vi "Main.vi"() -> ()   [LabVIEW 2013]
uses:
  <vilib>/Utility/sysdir.llb/System Directory Type.ctl
panel:
  out "Application:Kind":T1(ring)
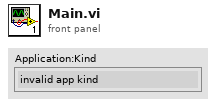
[diagram p1: front panel]
types:
  T1 = enum32{"invalid app kind", "Development System", "Run Time System", "Student Edition", "Embedded LabVIEW", "Evaluation", "Custom"}
  T2 = typedef "System Directory Type.ctl" = i32
  T3 = enum16{"open", "replace", "create", "open or create", "replace or create", "replace or create with confirmation"}
  T4 = cluster{"Missed Shots":dbl, "Over Truss With Catch":dbl, "Over the Truss Pass":dbl, "Defense?":string, "Can they pick up the ball?":string, "Can they catch?":string}
  T5 = cluster{"Autonomous?":string, "Did they start in \nthe goalie zone?":string, "Did they move?":string, "Was the goal lit?":string}
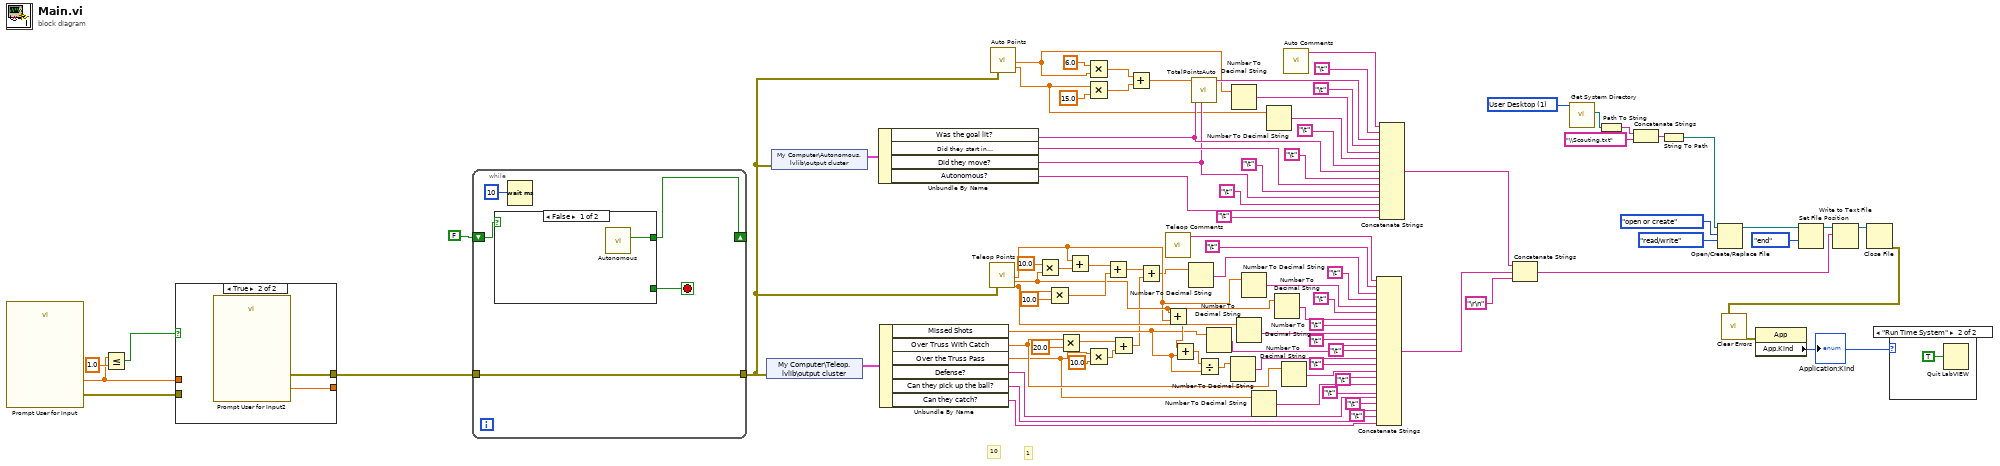
[diagram p0: block diagram]
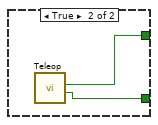
[diagram p4: hidden frame]
diagram:
  w80 = T2 1 items=["User Home"=0, "User Desktop"=1, "User Documents"=2, "User Application Data"=3, "User Preferences"=4, "User Temporary"=5, "Public Documents"=6, "Public Application Data"=7, "Public Preferences"=8, "Public Cache"=13, "System Core Libraries"=9, "System Installed Libraries"=10, "Application Files"=11, "Boot Volume Root"=12] ("system directory type")
  # "1"
  # "10"
  n1 = call "Prompt User for Input"() -> ("Team"=w76:dbl, "error out"=w75:errorcluster)  [unwired: 17 in, 1 out]
  n2 = Less Or Equal?(x=w76, y=1.0 ("x")) -> (x <= y?=w77:bool)
  n3 = case shown="True" w77 {
    tunnel: [w96 w98] -> _
    tunnel: w76 -> [w96 _]
    tunnel: w75 -> [w95 _]
    tunnel: [w95 w97] -> w74
    frame False {
    }
    frame True {
      n4 = call "Prompt User for Input2"() -> ("Team"=w98:dbl, "error out"=w97:errorcluster)  [unwired: 17 in, 1 out]
    }
  }
  n5 = while {
    shift-right: [w101] -> _
    shift-left: FALSE ("Boolean") -> [w102]
    tunnel: w74 -> [w99]
    tunnel: [w99] -> w71
    stop <- w100 stop-if-true
    n6 = case shown="False" w102 {
      tunnel: [w104 w105] -> w101
      tunnel: [_ w106] -> w100
      frame False {
        n7 = call "Autonomous.vi"() -> ("Switch To Teleop"=w104:bool)  [unwired: 10 in, 1 out]
      }
      frame True {
        n8 = call "Teleop.vi"() -> ("Stop program and write to file"=w106:bool, "SWITCH TO AUTONOMOUS 2"=w105:bool)  [unwired: 9 in, 1 out]
      }
    }
    n9 = Wait (ms)(milliseconds to wait=u32 10) -> ()  [unwired: 1 out]
  }
  n10 = shared-variable "My Computer\\Teleop.lvlib\\output cluster"(error in=w71) -> (w73:T4)  [unwired: 1 out]
  n11 = shared-variable "My Computer\\Autonomous.lvlib\\output cluster"(error in=w71) -> (w72:T5)  [unwired: 1 out]
  n12 = Unbundle By Name(w72) -> ("Was the goal lit?"=w58:string, "Did they start in \nthe goalie zone?"=w56:string, "Did they move?"=w54:string, "Autonomous?"=w52:string)
  n13 = Unbundle By Name(w73) -> ("Missed Shots"=w27:dbl, "Over Truss With Catch"=w16:dbl, "Over the Truss Pass"=w13:dbl, "Defense?"=w9:string, "Can they pick up the ball?"=w8:string, "Can they catch?"=w7:string)
  n14 = call "Teleop Points.vi"("Error In"=w71) -> ("Bottom Goal"=w30:dbl, "Top Goal"=w31:dbl, "Assists"=w38:dbl)  [unwired: 15 in, 1 out]
  n15 = call "Auto Points.vi"("Error In"=w71) -> ("Bottom Goal"=w50:dbl, "Top Goal"=w49:dbl)  [unwired: 16 in, 1 out]
  n16 = Multiply(x=10.0, y=w31) -> (x*y=w39:dbl)
  n17 = Multiply(x=w38, y=10.0) -> (x*y=w45:dbl)
  n18 = Multiply(x=w16, y=20.0) -> (x*y=w20:dbl)
  n19 = Add(x=w30, y=w39) -> (x+y=w44:dbl)
  n20 = Multiply(x=6.0, y=w50) -> (x*y=w63:dbl)
  n21 = Multiply(x=w49, y=15.0) -> (x*y=w61:dbl)
  n22 = Multiply(x=w13, y=10.0) -> (x*y=w21:dbl)
  n23 = Add(x=w44, y=w45) -> (x+y=w22:dbl)
  n24 = Add(x=w20, y=w21) -> (x+y=w18:dbl)
  n25 = Add(x=w63, y=w61) -> (x+y=w68:dbl)
  n26 = Add(x=w22, y=w18) -> (x+y=w17:dbl)
  n27 = call "Teleop Comments.vi"() -> ("Teleop Comments"=w48:string)  [unwired: 11 in]
  n28 = Add(x=w31, y=w30) -> (x+y=w29:dbl)
  n29 = Add(x=w29, y=w27) -> (x+y=w28:dbl)
  n30 = Number To Decimal String(number=w17) -> (decimal integer string=w42:string)  [unwired: 1 in]
  n31 = call "TotalPointsAuto.vi"("Did they move?"=w54, "Was the goal lit?"=w58, "input"=w68) -> ("Total Auto Points"=w65:string)  [unwired: 8 in]
  n32 = Divide(x=w28, y=w27) -> (x/y=w26:dbl)
  n33 = Number To Decimal String(number=w27) -> (decimal integer string=w32:string)  [unwired: 1 in]
  n34 = Number To Decimal String(number=w26) -> (decimal integer string=w25:string)  [unwired: 1 in]
  n35 = Number To Decimal String(number=w50) -> (decimal integer string=w62:string)  [unwired: 1 in]
  n36 = Number To Decimal String(number=w38) -> (decimal integer string=w34:string)  [unwired: 1 in]
  n37 = Number To Decimal String(number=w30) -> (decimal integer string=w40:string)  [unwired: 1 in]
  n38 = Number To Decimal String(number=w13) -> (decimal integer string=w11:string)  [unwired: 1 in]
  n39 = Number To Decimal String(number=w49) -> (decimal integer string=w60:string)  [unwired: 1 in]
  n40 = Number To Decimal String(number=w31) -> (decimal integer string=w36:string)  [unwired: 1 in]
  n41 = Number To Decimal String(number=w16) -> (decimal integer string=w14:string)  [unwired: 1 in]
  n42 = call "Auto Comments.vi"() -> ("Auto Comment"=w67:string)  [unwired: 11 in]
  n43 = Concatenate Strings(w48, "\t", w42, "\t", w40, "\t", w36, "\t", w34, "\t", w32, "\t", w25, "\t", w14, "\t", w11, "\t", w9, "\t", w8, "\t", w7) -> (w4:string)
  n44 = Concatenate Strings(w67, "\t", w65, "\t", w62, w60, "\t", w58, "\t", w56, "\t", w54, "\t", w52, "\t") -> (w3:string)
  n45 = Concatenate Strings(w3, w4, "\r\n") -> (w1:string)
  n46 = call <vilib>:"Get System Directory.vi"("system directory type"=w80) -> ("system directory"=w84:path)  [unwired: 10 in]
  n47 = Path To String(path=w84) -> (string=w83:string)
  n48 = Concatenate Strings(w83, "\\Scouting.txt" ("string")) -> (w82:string)
  n49 = String To Path(string=w82) -> (path=w79:path)
  n50 = Open/Create/Replace File(file path (use dialog)=w79, operation (0:open)=T3."open or create", access (0:read/write)=enum16{"read/write", "read-only", "write-only"}."read/write") -> (refnum out=w92:refnum<file>)  [unwired: 3 in, 2 out]
  n51 = Set File Position(refnum=w92, from (0:start)=enum16{"start", "end", "current"}."end") -> (refnum out=w93:refnum<file>)  [unwired: 2 in, 1 out]
  n52 = Write to Text File(file (use dialog)=w93, text=w1) -> (refnum out=w90:refnum<file>)  [unwired: 2 in, 2 out]
  n53 = Close File(refnum=w90) -> (error out=w85:errorcluster)  [unwired: 1 in, 1 out]
  n54 = call <vilib>:"Clear Errors.vi"("error in (no error)"=w85) -> ("error out"=w86:errorcluster)  [unwired: 6 in]
  n55 = property class="App"(error in=w86) -> ("App.Kind"=w87:T1)  [unwired: 1 in, 2 out]
  "Application:Kind" <- w87
  n56 = case shown="\"Run Time System\"" w87 {
    frame Default {
    }
    frame "Run Time System" {
      n57 = Quit LabVIEW(quit? (T)=TRUE) -> ()
    }
  }
